vi "Set Default Value.vi"(9 "Default C++ Value":string, 10 "Control Ref":refnum<vi>, 11 "Identity Writer in":refnum<class "Identity Writer.lvclass">) -> (1 "LabVIEW Default String":string, 2 "Control Ref Dup":refnum<vi>, 3 "Identity Writer out":refnum<class "Identity Writer.lvclass">)   [LabVIEW 2014, in "Identity Writer.lvclass"]
doc: "Copyright (c) 2016 Sze Howe Koh\n\nThis Source Code Form is subject to the terms of the Mozilla Public License, v. 2.0. If a copy of the MPL was not distributed with this file, You can obtain one at http://mozilla.org/MPL/2.0/."
uses:
  Identity Writer.lvclass
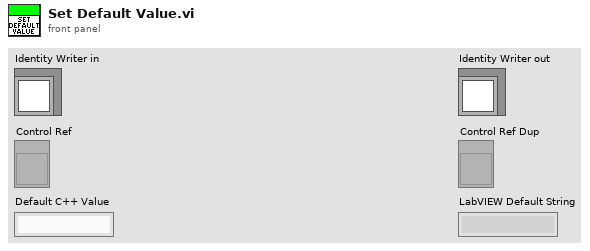
[diagram p1: front panel]
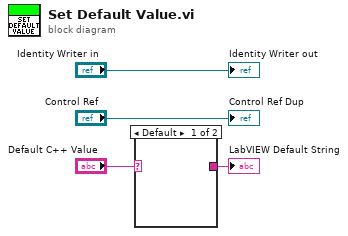
[diagram p0: block diagram]
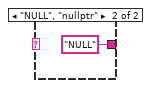
[diagram p2: hidden frame]
diagram:
  n1 = case shown="Default" "Default C++ Value" {
    tunnel: [_ "NULL"] -> w1
    frame Default {
    }
    frame "NULL", "nullptr" {
    }
  }
  "LabVIEW Default String" <- w1
  "Identity Writer out" <- "Identity Writer in"
  "Control Ref Dup" <- "Control Ref"
